vi "Mini Map Control Refernce.vi"(8 "Error In":errorcluster) -> (0 "Error Out":errorcluster, 3 "Mini Map Reference":refnum<k24>)   [LabVIEW 2014]
uses:
  C:/Robotic Systems/Products/Surveyor/Software/Ground Station/Data/Mapping DLL/GMap.NET.WindowsForms.dll
  Data/Mapping DLL/GMap.NET.WindowsForms.dll
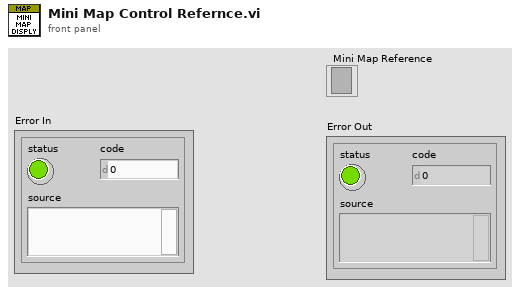
[diagram p1: front panel]
types:
  T1 = typedef "Mapping References.ctl" = cluster{"Main Map DLL Reference":refnum<k24>, "Main Map Control Reference":refnum<k24>, "Mini Map DLL Reference":refnum<k24>, "Mini Map Control Reference":refnum<k24>}
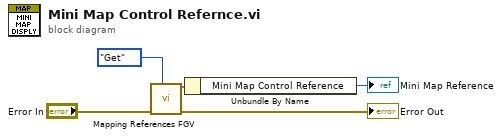
[diagram p0: block diagram]
diagram:
  n1 = call "Mapping References FGV.vi"("Method"=enum16{"Get", "Set"}."Get", "Error In"="Error In") -> ("Error Out"=→"Error Out":errorcluster, "Map References Out"=w2:T1)  [unwired: 8 in]
  n2 = Unbundle By Name(w2) -> ("Mini Map Control Reference"=→"Mini Map Reference":refnum<k24>)
